vi "AD5933_Reset (NI-845x I2C)(SubVI).vi"(7 "error in":errorcluster, 10 "NI-845x Config for I2C (in)":cluster{"i2c configuration":T1, "Refnum in":T2}) -> (0 "error out":errorcluster, 3 "NI-845x Config for I2C (out)":T3)   [LabVIEW 2017]
uses:
  <vilib>/ni845x/ni845x.llb/ni845xI2cConfiguration.ctl
  <vilib>/ni845x/ni845x.llb/ni845xControl.ctl
  TypeDefs/AD5933_Registers.ctl
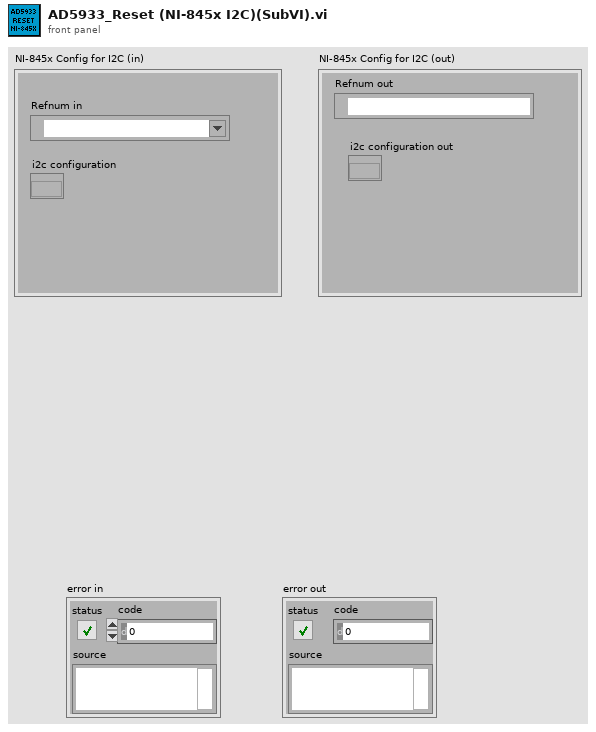
[diagram p1: front panel]
types:
  T1 = typedef "ni845xI2cConfiguration.ctl" = refnum<k20>
  T2 = typedef "ni845xControl.ctl" = refnum<k21>
  T3 = cluster{"i2c configuration out":T1, "Refnum out":T2}
  T4 = cluster{"Boolean array[0]":bool, "Reserved (0) [1]":bool, "Reserved (0) [2]":bool, "Externel system clock [3]":bool, "Reset[4]":bool, "Reserved (0) [5]":bool, "Reserved (0) [6]":bool, "Reserved (0) [7]":bool}
  T5 = typedef "AD5933_Registers.ctl" = u8
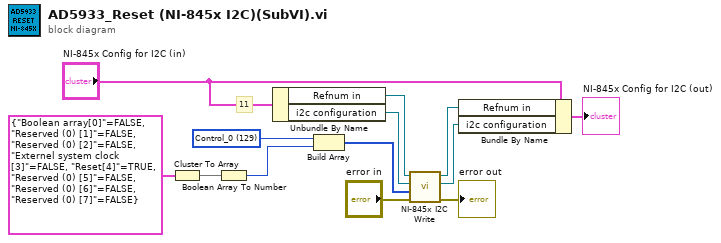
[diagram p0: block diagram]
diagram:
  w4 = T5 129 items=["Control_1"=128, "Control_0"=129, "StartFeq_2"=130, "StartFeq_1"=131, "StartFeq_0"=132, "FreqInc_2"=133, "FreqInc_1"=134, "FreqInc_0"=135, "NumOfInc_1"=136, "NumOfInc_0"=137, "NumOfSetCycl_1"=138, "NumOfSetCycl_0"=139, "Status"=143, "TempData_1"=146, "TempData_0"=147, "RealData_1"=148, "RealData_0"=149, "ImagData_1"=150, "ImagData_0"=151] ("Register")
  # "11"
  n1 = Cluster To Array(cluster=T4 {"Boolean array[0]"=FALSE, "Reserved (0) [1]"=FALSE, "Reserved (0) [2]"=FALSE, "Externel system clock [3]"=FALSE, "Reset[4]"=TRUE, "Reserved (0) [5]"=FALSE, "Reserved (0) [6]"=FALSE, "Reserved (0) [7]"=FALSE}) -> (array=w3:bool[])
  n2 = Boolean Array To Number(Boolean array=w3) -> (number=w1:u32)
  n3 = Unbundle By Name("NI-845x Config for I2C (in)") -> ("Refnum in"=w10:T2, "i2c configuration"=w9:T1)
  n4 = Build Array(w4, w1) -> (w5:u32[])
  n5 = call <vilib>:"NI-845x I2C Write.vi"("error in (no error)"="error in", "write data"=w5, "i2c configuration in"=w9, "device reference in"=w10) -> ("error out"=→"error out":errorcluster, "i2c configuration out"=w12:T1, "device reference out"=w11:T2)  [unwired: 5 in]
  n6 = Bundle By Name(cluster="NI-845x Config for I2C (in)", "Refnum in"=w11, "i2c configuration"=w12) -> (→"NI-845x Config for I2C (out)":cluster{"i2c configuration":T1, "Refnum in":T2})
